vi "DrawSpotMapSIMA.vi"(5 "x":dbl[](array[numeric]), 6 "Draw Mode":u16(ring) items=["Frame", "Paint", "Invert Frame", "Invert Paint"], 7 "error in (no error)":errorcluster, 8 "radius":i32, 9 "y":dbl[](array[numeric]), 10 "Image Dst":T1) -> (0 "error out":errorcluster, 2 "Spot Map":T1)   [LabVIEW 2009]
uses:
  <vilib>/vision/Image Controls.llb/IMAQ Image.ctl
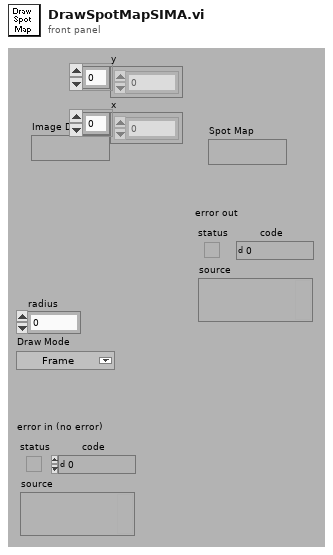
[diagram p1: front panel]
types:
  T1 = typedef "IMAQ Image.ctl" = refnum<image>
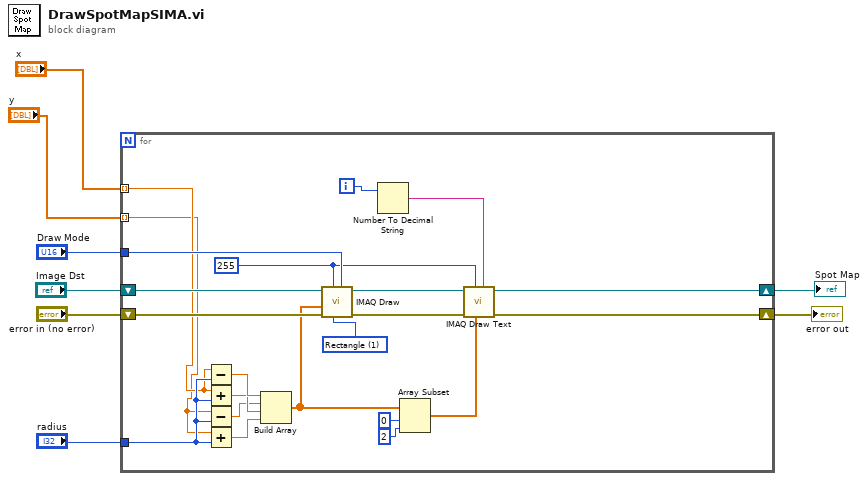
[diagram p0: block diagram]
diagram:
  n1 = for {
    shift-right: [w19] -> w7
    shift-left: "Image Dst" -> [w30]
    tunnel: "radius" -> [w27]
    tunnel: "Draw Mode" -> [w23]
    shift-right: [w11] -> w5
    shift-left: "error in (no error)" -> [w22]
    tunnel: "x" -> [w10] mode=indexing
    tunnel: "y" -> [w9] mode=indexing
    i -> [w16]
    w18 = 255
    w24 = u16 1 items=["Line", "Rectangle", "Oval"] ("Shape to draw")
    n2 = Subtract(x=w10, y=w27) -> (x-y=w29:dbl)
    n3 = Add(x=w10, y=w27) -> (x+y=w28:dbl)
    n4 = Subtract(x=w9, y=w27) -> (x-y=w26:dbl)
    n5 = Add(x=w9, y=w27) -> (x+y=w25:dbl)
    n6 = Build Array(w29, w26, w28, w25) -> (w15:dbl[])
    n7 = call "IMAQ Draw"("Draw Mode"=w23, "Shape to draw"=w24, "Pixel Color"=w18, "error in (no error)"=w22, "Coordinates"=w15, "Image Src"=w30) -> ("error out"=w20:errorcluster, "Image Dst Out"=w21:T1)  [unwired: 4 in]
    n8 = Number To Decimal String(number=w16) -> (decimal integer string=w17:string)  [unwired: 1 in]
    n9 = Array Subset(array=w15, index=0, length=2) -> (w14:dbl[])
    n10 = call "IMAQ Draw Text"("String"=w17, "Insertion Point"=w14, "Color"=w18, "error in (no error)"=w20, "Image Src"=w21) -> ("error out"=w11:errorcluster, "Image Dst Out"=w19:T1)  [unwired: 3 in, 2 out]
  }
  "Spot Map" <- w7
  "error out" <- w5
